vi "Example - Insert into a Table.vi"() -> ()   [LabVIEW 2013]
doc: "This example opens a connection to a database specified by the Connection string (replace the DNS name with your database) inserts a new row into the table \"myOtherTable\" (replace the SQL string with your own SQL query)."
panel:
  out "error out":errorcluster
  in  "Command Text":string="INSERT INTO myOtherTable\n (Location, Temp, Humidity)\nVALUES ('Austin', 102, 95);"
  in  "ConnectionString":string="DSN=myDB;"
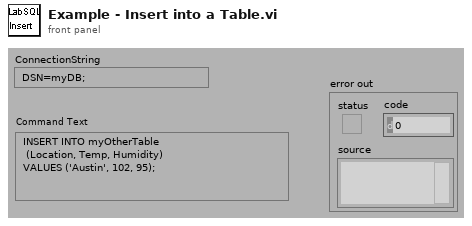
[diagram p1: front panel]
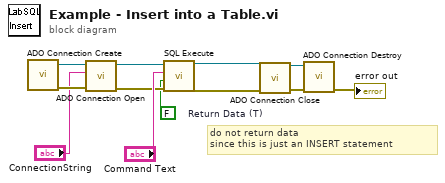
[diagram p0: block diagram]
diagram:
  w1 = FALSE  # Return Data (T)
  # "do not return data\nsince this is just an INSERT statement"
  n1 = call "ADO Connection Create.vi"() -> ("error out"=w11:errorcluster, "ADODB._Connection Out"=w12:refnum<k7>)  [unwired: 10 in]
  n2 = call "ADO Connection Open.vi"("error in (no error)"=w11, "ConnectionString"="ConnectionString", "ADODB._Connection In"=w12) -> ("error out"=w7:errorcluster, "ADODB._Connection Out"=w9:refnum<k7>)  [unwired: 7 in]
  n3 = call "SQL Execute.vi"("error in (no error)"=w7, "Return Data (T)"=w1, "Command Text"="Command Text", "ADODB._Connection In"=w9) -> ("error out"=w6:errorcluster, "ADODB._Connection Out"=w5:refnum<k7>)  [unwired: 4 in, 2 out]
  n4 = call "ADO Connection Close.vi"("error in (no error)"=w6, "ADODB._Connection In"=w5) -> ("error out"=w4:errorcluster, "ADODB._Connection Out"=w3:refnum<k7>)  [unwired: 8 in]
  n5 = call "ADO Connection Destroy.vi"("error in (no error)"=w4, "ADODB._Connection In"=w3) -> ("error out"=→"error out":errorcluster)  [unwired: 9 in]
